vi "myRIO__TCP_constants_byteRange_packet__checkRange.vi"(11 "input_byte":u8) -> (0 "output_packet_end":bool, 1 "output_packet_start":bool, 3 "output_packet":bool)   [LabVIEW 2014]
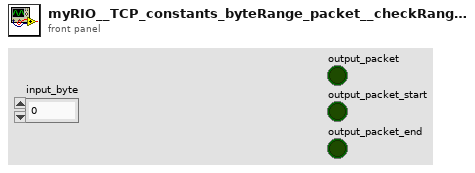
[diagram p1: front panel]
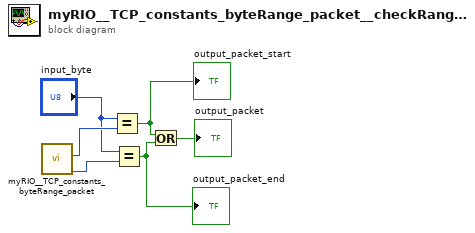
[diagram p0: block diagram]
diagram:
  n1 = call "myRIO__TCP_constants_byteRange_packet.vi"() -> ("output_end_byte"=w5:u8, "output_start_byte"=w6:u8)  [unwired: 8 in, 2 out]
  n2 = Equal?(x="input_byte", y=w6) -> (x = y?=w3:bool)
  "output_packet_start" <- w3
  n3 = Equal?(x="input_byte", y=w5) -> (x = y?=w2:bool)
  "output_packet_end" <- w2
  n4 = Or(x=w3, y=w2) -> (x .or. y?=→"output_packet":bool)
